vi "12.1-TopHat&GrayMorphReconstruct.vi"() -> ()   [LabVIEW 2016]
doc: "This example shows how to use the Edge Tool in NI Vision. The Edge Tool finds edges (or sharp transitions in the pixels values) along a given line or ROI profile. The Edge Tool is a precursor function to many of the gauging and inspection tasks. For example, the location of the edges found along a line profile across an object can interpreted as the boundaries of the object whose dimensions have to be measured for a gauging application or the presence of a crack in the surface of an object for an inspection application."
uses:
  <vilib>/vision/NI_Vision_Development_Module.lvlib
panel:
  out "Src":T1(plugin-control)
  in  "Hexa Pixel?":bool
  in  "Operation":u16(ring)=8 items=["AutoM", "Close", "Dilate", "Erode", "Gradient", "Gradient out", "Gradient in", "Hit miss", "Open", "PClose", "POpen", "Thick", "Thin"]
  out "Dst":T1(plugin-control)
  in  "Stop":bool
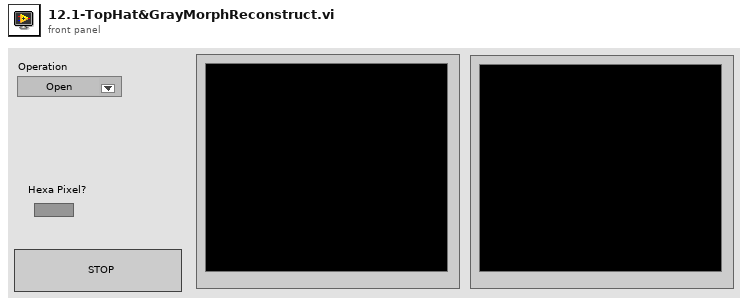
[diagram p1: front panel]
types:
  T1 = typedef "IMAQ Image.ctl" = refnum<image>
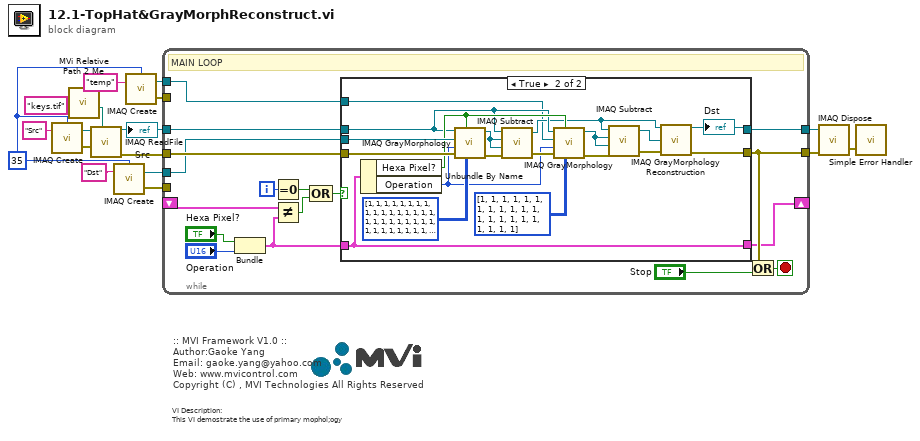
[diagram p0: block diagram]
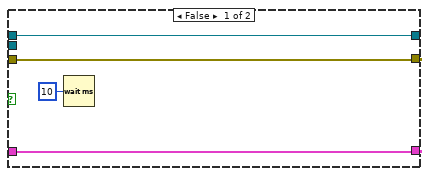
[diagram p2: hidden frame]
diagram:
  w5 = 35 ("Border Size")
  # "VI Description:\nThis VI demostrate the use of primary mophol;ogy"
  # ":: MVI Framework V1.0 ::\nAuthor:Gaoke Yang\nEmail: gaoke.yang@yahoo.com\nWeb: www.mvicontrol.com\nCopyright (C) , MVI Technologies All Rights Reserved"
  n1 = call "IMAQ Create"("Border Size"=w5, "Image Name"="Src") -> ("New Image"=w16:T1, "error out"=w15:errorcluster)  [unwired: 3 in]
  n2 = call "MVi Relative Path 2 Me.vi"("Relative Path"="keys.tif" ("name or relative path")) -> ("Appended Dir"=w12:path)  [unwired: 5 in, 1 out]
  n3 = call "IMAQ ReadFile"("File Path"=w12, "error in (no error)"=w15, "Image"=w16) -> ("error out"=w6:errorcluster, "Image Out"=w7:T1)  [unwired: 4 in, 3 out]
  "Src" <- w7
  n4 = call "IMAQ Create"("Border Size"=w5, "Image Name"="Dst") -> ("New Image"=w9:T1, "error out"=w8:errorcluster)  [unwired: 3 in]
  n5 = call "IMAQ Create"("Border Size"=w5, "Image Name"="temp") -> ("New Image"=w2:T1, "error out"=w3:errorcluster)  [unwired: 3 in]
  n6 = while "MAIN LOOP" {
    tunnel: w7 -> [w33]
    tunnel: w6 -> [w34]
    tunnel: [w30] -> w14
    shift-right: [w27] -> _
    shift-left: _ -> [w24]
    tunnel: w9 -> [w22]
    tunnel: w8 -> [_]
    tunnel: w3 -> [_]
    tunnel: w2 -> [w19]
    tunnel: [w18] -> w1
    i -> [w29]
    stop <- w31 stop-if-true
    # "MAIN LOOP"
    n7 = Bundle("Hexa Pixel?"="Hexa Pixel?", "Operation"="Operation") -> (w25:cluster{"Hexa Pixel?":bool, "Operation":u16})  [unwired: 1 in]
    n8 = Equal To 0?(x=w29) -> (x = 0?=w26:bool)
    n9 = Not Equal?(x=w24, y=w25) -> (x != y?=w23:bool)
    n10 = Compound Arithmetic op=OR(w26, w23) -> (w28:bool)
    n11 = case shown="True" w28 {
      tunnel: w34 -> [w38 w56]
      tunnel: w33 -> [w35 w48]
      tunnel: [w38 w41] -> w30
      tunnel: [w36 w57] -> w27
      tunnel: w25 -> [w36 w57]
      tunnel: w22 -> [_ w55]
      tunnel: w19 -> [_ w42]
      tunnel: [w35 w39] -> w18
      frame False {
        n12 = Wait (ms)(milliseconds to wait=u32 10) -> ()  [unwired: 1 out]
      }
      frame True {
        n13 = Unbundle By Name(w57) -> ("Hexa Pixel?"=w52:bool, "Operation"=w43:u16)
        n14 = call "IMAQ GrayMorphology"("Structuring Element"=i32[][] [[1, 1, 1, 1, 1, 1, 1, 1, 1, 1, 1, 1, 1, 1, 1, 1, 1, 1, 1, 1, 1, 1, 1, 1, 1, 1, 1, 1, 1, 1, 1, 1, 1, 1, 1, 1, 1, 1, 1, 1, 1, 1, 1, 1, 1, 1, 1, 1, 1, 1, 1, 1, 1, 1, 1, 1, 1, 1, 1, 1, 1, 1, 1, 1, 1, 1, 1, 1, 1, 1, 1, 1]], "Square/Hexa (Square)"=w52, "error in (no error)"=w56, "Operation"=w43, "Image Dst"=w55, "Image Src"=w48) -> ("error out"=w51:errorcluster, "Image Dst Out"=w50:T1)  [unwired: 4 in]
        n15 = call "IMAQ Subtract"("Image Src A"=w48, "Image Dst"=w50, "Image Src B"=w50, "error in (no error)"=w51) -> ("Image Dst Out"=w46:T1, "error out"=w49:errorcluster)  [unwired: 3 in]
        n16 = call "IMAQ GrayMorphology"("Structuring Element"=i32[][] [[1], [1], [1], [1], [1], [1], [1], [1], [1], [1], [1], [1], [1], [1], [1], [1], [1], [1], [1], [1], [1], [1]], "Square/Hexa (Square)"=w52, "error in (no error)"=w49, "Operation"=w43, "Image Dst"=w42, "Image Src"=w48) -> ("error out"=w53:errorcluster, "Image Dst Out"=w45:T1)  [unwired: 4 in]
        n17 = call "IMAQ Subtract"("Image Src A"=w46, "Image Dst"=w45, "Image Src B"=w45, "error in (no error)"=w53) -> ("Image Dst Out"=w40:T1, "error out"=w47:errorcluster)  [unwired: 3 in]
        n18 = call "IMAQ GrayMorphology Reconstruction"("Image Src"=w46, "Image Marker"=w40, "error in (no error)"=w47) -> ("Image Dst Out"=w39:T1, "error out"=w41:errorcluster)  [unwired: 11 in]
        "Dst" <- w39
      }
    }
    n19 = Or(x=w30, y="Stop") -> (x .or. y?=w31:bool)
  }
  n20 = call "IMAQ Dispose"("Image"=w1, "error in (no error)"=w14) -> ("error out"=w11:errorcluster)  [unwired: 4 in]
  n21 = call <vilib>:"Simple Error Handler.vi"("error in (no error)"=w11) -> ()  [unwired: 4 in, 5 out]
